vi "DAQ_CounterTrigger_DO_AO_2DAQ.vi"(8 "error in (no error)":errorcluster) -> (0 "error out":errorcluster)   [LabVIEW 2025]
uses:
  SubVIs/State_Machine_Ctrl.ctl
  <vilib>/DAQmx/write.llb/DAQmx Write (Digital 1D Wfm NChan NSamp).vi
  <vilib>/DAQmx/write.llb/DAQmx Write (Analog 1D Wfm NChan NSamp).vi
  <vilib>/Waveform/DWDTOps.llb/DWDT Uncompress Digital.vi
  <vilib>/DAQmx/miscellaneous.llb/DAQmx Fill In Error Info.vi
  <resource>/objmgr/daqmx.rc
panel:
  in  "Z":bool=TRUE
  in  "AO Z":tag="USB-6211/ao1"
  out "AO WF":waveform(dbl)[](graph)=[{"t0"=timestamp(0 s since 1904-01-01), "dt"=0.0001, "Y"=array[9000 elements]}, {"t0"=timestamp(0 s since 1904-01-01), "dt"=0.0001, "Y"=array[9000 elements]}, {"t0"=timestamp(0 s since 1904-01-01), "dt"=0.0001, "Y"=array[9000 elements]}, {"t0"=timestamp(0 s since 1904-01-01), "dt"=0.0001, "Y"=array[9000 elements]}]
  out "DO WF":digitalwaveform[](graph)=[{"t0"=timestamp(0 s since 1904-01-01), "dt"=0.0001, "Y"={"transitions"=[], "data"=array9000x1[9000 elements]}}, {"t0"=timestamp(0 s since 1904-01-01), "dt"=0.0001, "Y"={"transitions"=[], "data"=array9000x1[9000 elements]}}, {"t0"=timestamp(0 s since 1904-01-01), "dt"=0.0001, "Y"={"transitions"=[], "data"=array9000x1[9000 elements]}}, {"t0"=timestamp(0 s since 1904-01-01), "dt"=0.0001, "Y"={"transitions"=[], "data"=array9000x1[9000 elements]}}]
  in  "Polar | ON/OFF":bool=TRUE
  in  "AO | %":dbl[](array[slide])=[9.734513274336283, 23.008849557522126, 41.5929203539823, 65.48672566371681] min=0.0 max=100.0 step=1.0 scale=0.0..100.0
  in  "AO | ON/OFF":bool[](array[boolean])=[TRUE, TRUE, TRUE, TRUE]
  in  "AO Laser":tag="USB-6363/ao0:3"
  in  "AO pockels":tag="USB-6211/ao0"
  in  "DO | ON/OFF":bool[](array[boolean])=[TRUE, TRUE, TRUE, TRUE, TRUE]
  in  "Pre-activation time (s)":dbl=0.03
  in  "Start":bool
  in  "Timing source":tag="OnboardClock"
  in  "Readout time (s)":dbl=0.02
  in  "Exposure time (s)":dbl=0.05
  in  "DO":tag="USB-6363/port0/line0:4"
  in  "Counter":tag="USB-6363/ctr0"
  in  "Stop":bool
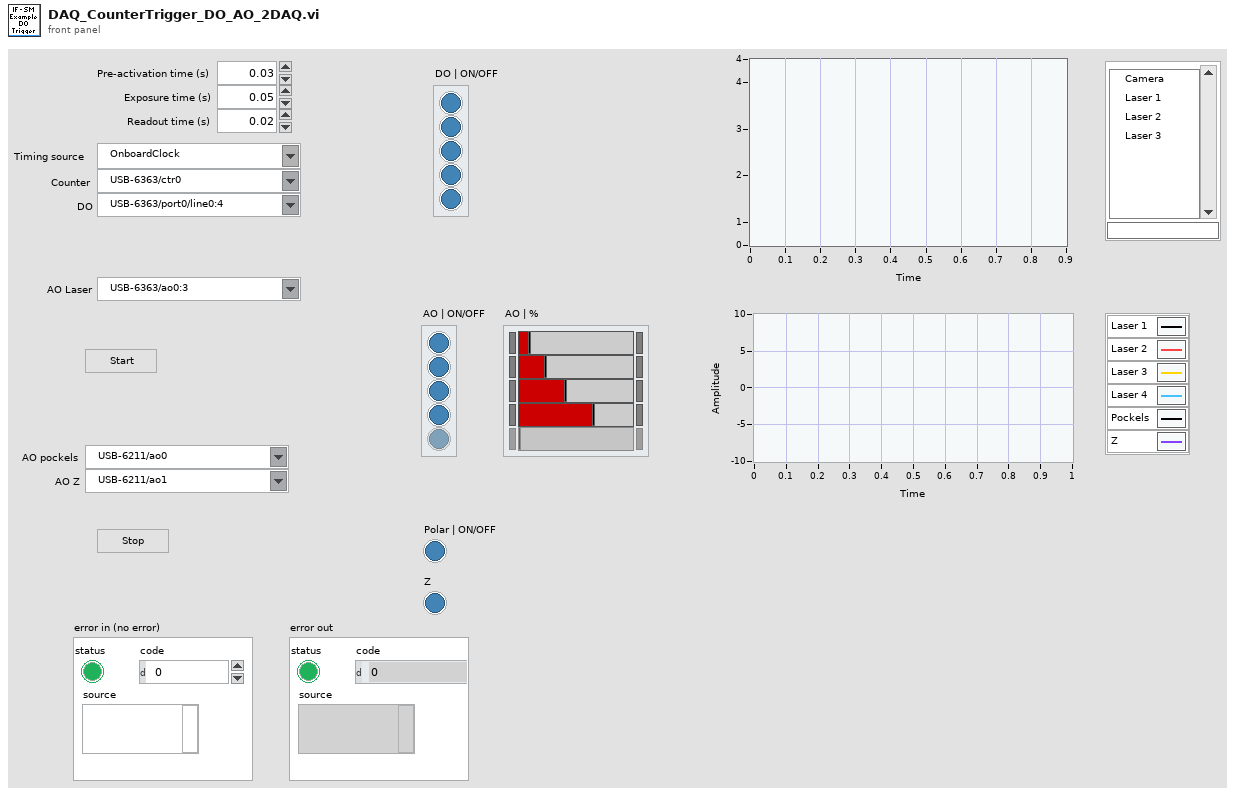
[diagram p1: front panel]
types:
  T1 = typedef "State_Machine_Ctrl.ctl" = enum16{"Initialize", "Wait for Event", "Setup_DAQ", "Create WF", "Generate WF", "Stop"}
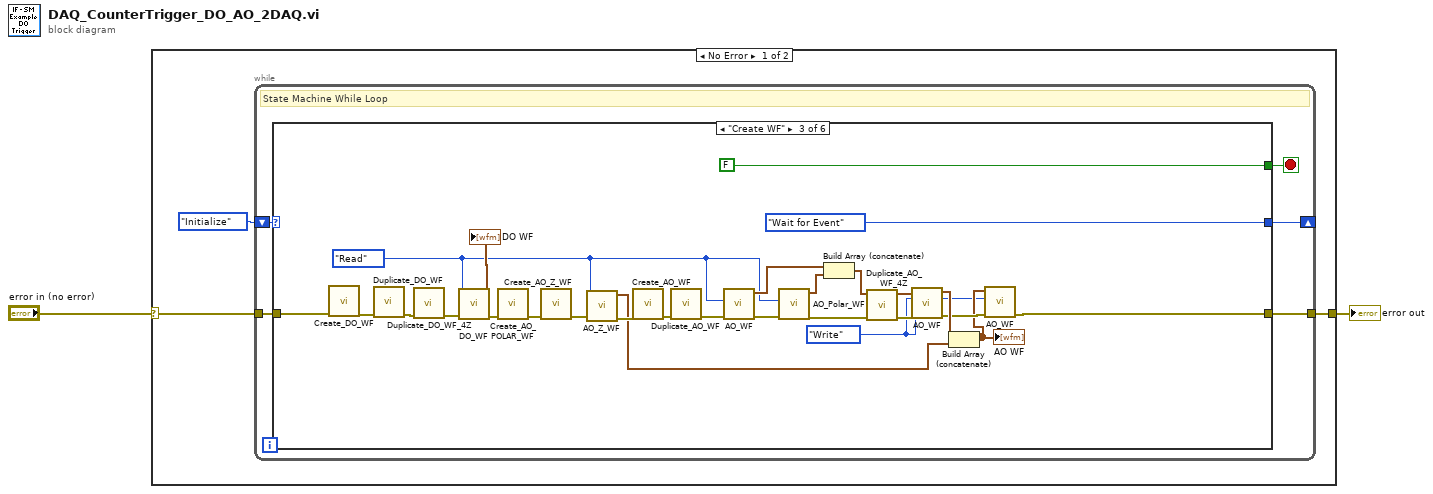
[diagram p0: block diagram]
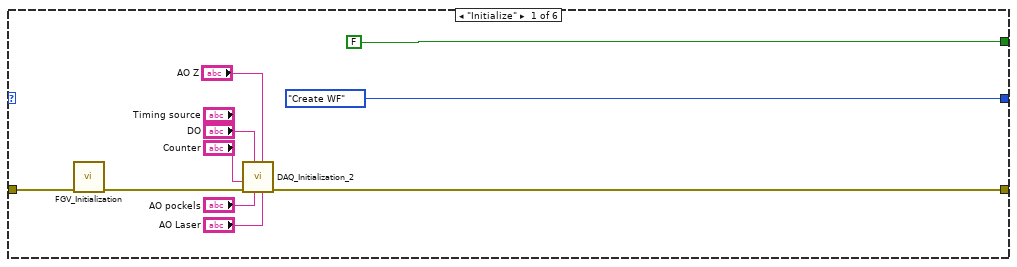
[diagram p2: hidden frame]
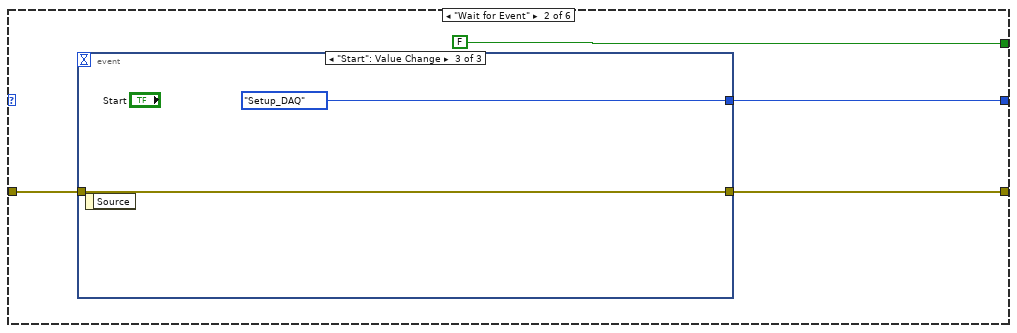
[diagram p3: hidden frame]
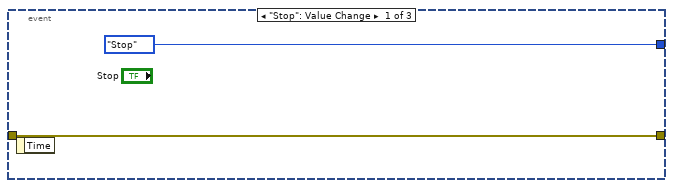
[diagram p4: hidden frame]
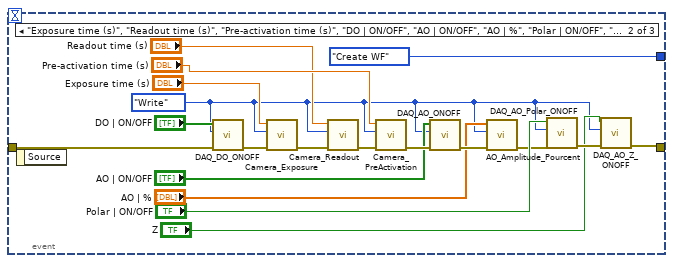
[diagram p5: hidden frame]
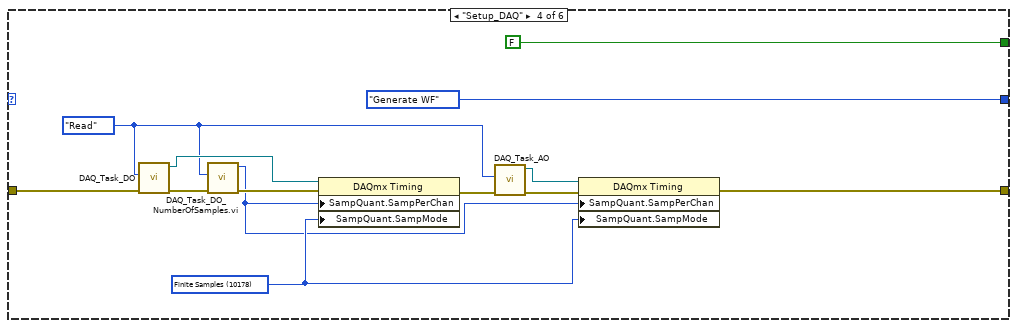
[diagram p6: hidden frame]
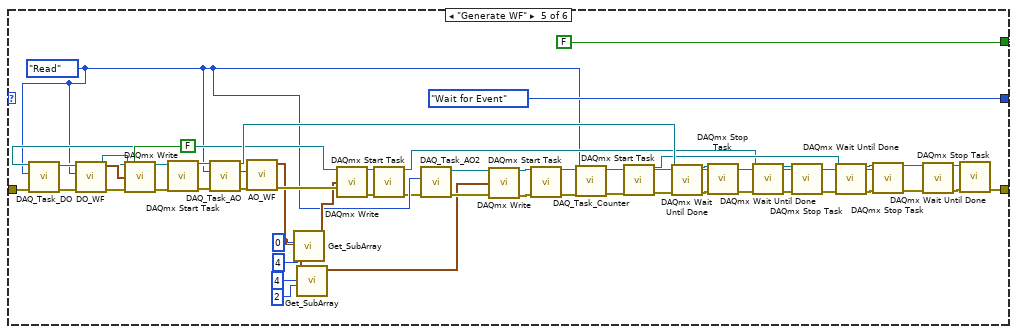
[diagram p7: hidden frame]
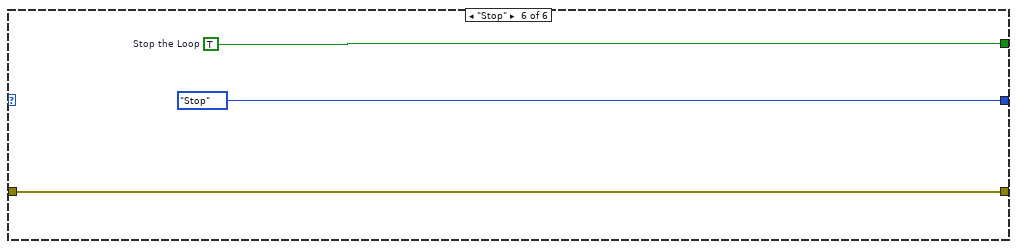
[diagram p8: hidden frame]
diagram:
  n1 = case shown="No Error" "error in (no error)" {
    selector: "error in (no error)" -> [w4 w140]
    tunnel: [w3 w140] -> w2
    frame No Error {
      n2 = while {
        shift-right: [w9] -> _
        shift-left: State_Machine_Ctrl."Initialize" ("Initial State") -> [w10]
        tunnel: w4 -> [w7]
        tunnel: [w6] -> w3
        stop <- w8 stop-if-true
        # "State Machine While Loop"
        n3 = case "State Machine Case Structure" shown="\"Create WF\"" w10 {
          tunnel: [State_Machine_Ctrl."Create WF" ("Initial State") w24 State_Machine_Ctrl."Wait for Event" ("Initial State") State_Machine_Ctrl."Generate WF" ("Initial State") State_Machine_Ctrl."Wait for Event" ("Initial State") State_Machine_Ctrl."Stop" ("Initial State")] -> w9
          tunnel: [FALSE ("Stop the Loop") FALSE ("Stop the Loop") FALSE ("Stop the Loop") FALSE ("Stop the Loop") FALSE ("Stop the Loop") w139] -> w8
          tunnel: w7 -> [w18 w22 w72 w85 w133 w137]
          tunnel: [w19 w21 w50 w82 w107 w137] -> w6
          frame "Initialize" {
            # "Initialize - In this example, the only initialization required is to specify that the next state for the state machine is \"Wait for Event\"."
            n4 = call "FGV_Initialization.vi"("error in (no error)"=w18) -> ("error out"=w17:errorcluster)  [unwired: 10 in]
            n5 = call "DAQ_Initialization_2.vi"("AO Lasers"="AO Laser", "AO Z"="AO Z", "AO Pockels"="AO pockels", "DO"="DO", "error in (no error)"=w17, "Counter"="Counter") -> ("error out"=w19:errorcluster)  [unwired: 5 in]
          }
          frame "Wait for Event" {
            # "Wait for Event - An Event Structure is used to monitor the user interface for events. In each frame of the Event Structure, the next state of the state machine is specified based on which button was pressed."
            n6 = event shown="[2] \"Start\": Value Change" {
              selector: _ -> [_ _ _]
              dyn-events: _ -> [_ _ _]
              timeout: _ -> [_ _ _]
              tunnel: [State_Machine_Ctrl."Stop" ("Initial State") State_Machine_Ctrl."Create WF" ("Initial State") State_Machine_Ctrl."Setup_DAQ" ("Initial State")] -> w24
              tunnel: w22 -> [w25 w41 w46]
              tunnel: [w25 w29 w46] -> w21
              event "Stop": Value Change {
                n7 = event-data() -> ()  [unwired: 1 in, 1 out]
              }
              event "Exposure time (s)", "Readout time (s)", "Pre-activation time (s)", "DO | ON/OFF", "AO | ON/OFF", "AO | %", "Polar | ON/OFF", "Z": Value Change {
                w27 = enum16{"Write", "Read"}."Write" ("Action")
                n8 = event-data() -> ()  [unwired: 1 in, 1 out]
                n9 = call "DAQ_DO_ONOFF.vi"("error in"=w41, "Action"=w27, "DO | ON/OFF"="DO | ON/OFF") -> ("error out"=w44:errorcluster)  [unwired: 7 in, 1 out]
                n10 = call "Camera_Exposure.vi"("error in"=w44, "Action"=w27, "Exposure (s)"="Exposure time (s)") -> ("error out"=w43:errorcluster)  [unwired: 7 in, 1 out]
                n11 = call "Camera_Readout.vi"("error in"=w43, "Action"=w27, "Camera_Readout"="Readout time (s)") -> ("error out"=w42:errorcluster)  [unwired: 7 in, 1 out]
                n12 = call "Camera_PreActivation.vi"("error in"=w42, "Action"=w27, "Camera_PreActivation"="Pre-activation time (s)") -> ("error out"=w36:errorcluster)  [unwired: 7 in, 1 out]
                n13 = call "DAQ_AO_ONOFF.vi"("error in"=w36, "Action"=w27, "AO | ON/OFF"="AO | ON/OFF") -> ("error out"=w34:errorcluster)  [unwired: 7 in, 1 out]
                n14 = call "AO_Amplitude_Pourcent.vi"("error in"=w34, "Action"=w27, "AO | %"="AO | %") -> ("error out"=w31:errorcluster)  [unwired: 7 in, 1 out]
                n15 = call "DAQ_AO_Polar_ONOFF.vi"("error in"=w31, "Action"=w27, "ON / OFF"="Polar | ON/OFF") -> ("error out"=w30:errorcluster)  [unwired: 7 in, 1 out]
                n16 = call "DAQ_AO_Z_ONOFF.vi"("error in"=w30, "Action"=w27, "ON / OFF"="Z") -> ("error out"=w29:errorcluster)  [unwired: 7 in, 1 out]
              }
              event "Start": Value Change {
                n17 = event-data() -> ()  [unwired: 1 in, 1 out]
              }
            }
          }
          frame "Create WF" {
            w48 = enum16{"Write", "Read"}."Write" ("Action")
            w63 = enum16{"Write", "Read"}."Read" ("Action")
            n18 = call "Create_DO_WF.vi"("error in"=w72) -> ("error out"=w71:errorcluster)  [unwired: 10 in]
            n19 = call "Duplicate_DO_WF.vi"("error in"=w71) -> ("error out"=w60:errorcluster)  [unwired: 10 in]
            n20 = call "Duplicate_DO_WF_4Z.vi"("error in"=w60) -> ("error out"=w59:errorcluster)  [unwired: 10 in]
            n21 = call "DO_WF.vi"("error in"=w59, "Action"=w63) -> ("error out"=w58:errorcluster, "Digital WF"=→"DO WF":digitalwaveform[])  [unwired: 8 in]
            n22 = call "Create_AO_POLAR_WF.vi"("error in"=w58) -> ("error out"=w64:errorcluster)  [unwired: 10 in]
            n23 = call "Create_AO_Z_WF.vi"("error in"=w64) -> ("error out"=w62:errorcluster)  [unwired: 10 in]
            n24 = call "AO_Z_WF.vi"("error in"=w62, "Action"=w63) -> ("error out"=w61:errorcluster, "AO Z WF"=w53:waveform(dbl))  [unwired: 8 in]
            n25 = call "Create_AO_WF.vi"("error in"=w61) -> ("error out"=w69:errorcluster)  [unwired: 10 in]
            n26 = call "Duplicate_AO_WF.vi"("error in (no error)"=w69) -> ("error out"=w68:errorcluster)  [unwired: 10 in]
            n27 = call "AO_WF.vi"("error in"=w68, "Action"=w63) -> ("error out"=w70:errorcluster, "AO WF"=w66:waveform(dbl)[])  [unwired: 8 in]
            n28 = call "AO_Polar_WF.vi"("error in"=w70, "Action"=w63) -> ("error out"=w54:errorcluster, "AO Poalr WF"=w65:waveform(dbl))  [unwired: 8 in]
            n29 = Build Array (concatenate)(w66, w65) -> (w57:waveform(dbl)[])
            n30 = call "Duplicate_AO_WF_4Z.vi"("error in (no error)"=w54, "AO WF"=w57) -> ("error out"=w55:errorcluster, "AO WF 2"=w56:waveform(dbl)[])  [unwired: 8 in]
            n31 = call "AO_WF.vi"("error in"=w55, "Action"=w48, "AO WF"=w56) -> ("error out"=w51:errorcluster, "AO WF"=w52:waveform(dbl)[])  [unwired: 7 in]
            n32 = Build Array (concatenate)(w52, w53) -> (w49:waveform(dbl)[])
            "AO WF" <- w49
            n33 = call "AO_WF.vi"("error in"=w51, "Action"=w48, "AO WF"=w49) -> ("error out"=w50:errorcluster)  [unwired: 7 in, 1 out]
          }
          frame "Setup_DAQ" {
            w79 = 10178 items=["Finite Samples"=10178, "Continuous Samples"=10123, "Hardware Timed Single Point"=12522] ("SampQuant.SampMode")
            w78 = enum16{"Write", "Read"}."Read" ("Action")
            n34 = call "DAQ_Task_DO.vi"("error in"=w85, "Action"=w78) -> ("error out"=w77:errorcluster, "DAQ_Task_DO"=w84:refnum<k21>)  [unwired: 8 in]
            n35 = call "DAQ_Task_DO_NumberOfSamples.vi.vi"("error in"=w77, "Action"=w78) -> ("error out"=w76:errorcluster, "Samples"=w75:u32)  [unwired: 8 in]
            n36 = property class="DAQmx Timing"(reference=w84, error in=w76, "SampQuant.SampPerChan"=w75, "SampQuant.SampMode"=w79) -> (error out=w80:errorcluster)  [unwired: 1 out]
            n37 = call "DAQ_Task_AO.vi"("error in"=w80, "Action"=w78) -> ("error out"=w83:errorcluster, "DAQ_Task_AO"=w81:refnum<k21>)  [unwired: 8 in]
            n38 = property class="DAQmx Timing"(reference=w81, error in=w83, "SampQuant.SampPerChan"=w75, "SampQuant.SampMode"=w79) -> (error out=w82:errorcluster)  [unwired: 1 out]
          }
          frame "Generate WF" {
            w97 = enum16{"Write", "Read"}."Read" ("Action")
            n39 = call "DAQ_Task_DO.vi"("error in"=w133, "Action"=w97) -> ("error out"=w120:errorcluster, "DAQ_Task_DO"=w132:refnum<k21>)  [unwired: 8 in]
            n40 = call "DO_WF.vi"("error in"=w120, "Action"=w97) -> ("error out"=w119:errorcluster, "Digital WF"=w121:digitalwaveform[])  [unwired: 8 in]
            n41 = call-poly <vilib>:"DAQmx Write.vi"("task/channels in"=w132, "auto start"=FALSE, "data"=w121, "error in"=w119) -> ("task out"=w131:refnum<k21>, "error out"=w134:errorcluster)  [unwired: 9 in, 1 out]
            n42 = call <vilib>:"DAQmx Start Task.vi"("task/channels in"=w131, "error in"=w134) -> ("task out"=w125:refnum<k21>, "error out"=w101:errorcluster)  [unwired: 12 in]
            n43 = call "DAQ_Task_AO.vi"("error in"=w101, "Action"=w97) -> ("error out"=w114:errorcluster, "DAQ_Task_AO"=w113:refnum<k21>)  [unwired: 8 in]
            n44 = call "AO_WF.vi"("error in"=w114, "Action"=w97) -> ("error out"=w112:errorcluster, "AO WF"=w91:waveform(dbl)[])  [unwired: 8 in]
            n45 = call "Get_SubArray.vi"("length"=4, "index"=0, "AO WF"=w91) -> ("Sub array"=w99:waveform(dbl)[])  [unwired: 8 in]
            n46 = call "Get_SubArray.vi"("length"=2, "index"=4, "AO WF"=w91) -> ("Sub array"=w90:waveform(dbl)[])  [unwired: 8 in]
            n47 = call-poly <vilib>:"DAQmx Write.vi"("task/channels in"=w113, "data"=w99, "error in"=w112) -> ("task out"=w111:refnum<k21>, "error out"=w110:errorcluster)  [unwired: 10 in, 1 out]
            n48 = call <vilib>:"DAQmx Start Task.vi"("task/channels in"=w111, "error in"=w110) -> ("task out"=w109:refnum<k21>, "error out"=w94:errorcluster)  [unwired: 12 in]
            n49 = call "DAQ_Task_AO2.vi"("error in"=w94, "Action"=w97) -> ("error out"=w100:errorcluster, "DAQ_Task_AO"=w105:refnum<k21>)  [unwired: 8 in]
            n50 = call-poly <vilib>:"DAQmx Write.vi"("task/channels in"=w105, "data"=w90, "error in"=w100) -> ("task out"=w104:refnum<k21>, "error out"=w103:errorcluster)  [unwired: 10 in, 1 out]
            n51 = call <vilib>:"DAQmx Start Task.vi"("task/channels in"=w104, "error in"=w103) -> ("task out"=w102:refnum<k21>, "error out"=w95:errorcluster)  [unwired: 12 in]
            n52 = call "DAQ_Task_Counter.vi"("error in"=w95, "Action"=w97) -> ("error out"=w96:errorcluster, "DAQ_Task_Counter"=w130:refnum<k21>)  [unwired: 8 in]
            n53 = call <vilib>:"DAQmx Start Task.vi"("task/channels in"=w130, "error in"=w96) -> ("task out"=w123:refnum<k21>, "error out"=w122:errorcluster)  [unwired: 12 in]
            n54 = call <vilib>:"DAQmx Wait Until Done.vi"("task/channels in"=w125, "error in"=w122) -> ("task out"=w124:refnum<k21>, "error out"=w126:errorcluster)  [unwired: 12 in]
            n55 = call <vilib>:"DAQmx Stop Task.vi"("task/channels in"=w124, "error in"=w126) -> ("error out"=w117:errorcluster)  [unwired: 12 in, 1 out]
            n56 = call <vilib>:"DAQmx Wait Until Done.vi"("task/channels in"=w109, "error in"=w117) -> ("task out"=w115:refnum<k21>, "error out"=w118:errorcluster)  [unwired: 12 in]
            n57 = call <vilib>:"DAQmx Stop Task.vi"("task/channels in"=w115, "error in"=w118) -> ("error out"=w116:errorcluster)  [unwired: 12 in, 1 out]
            n58 = call <vilib>:"DAQmx Wait Until Done.vi"("task/channels in"=w123, "error in"=w116) -> ("task out"=w128:refnum<k21>, "error out"=w127:errorcluster)  [unwired: 12 in]
            n59 = call <vilib>:"DAQmx Stop Task.vi"("task/channels in"=w128, "error in"=w127) -> ("error out"=w106:errorcluster)  [unwired: 12 in, 1 out]
            n60 = call <vilib>:"DAQmx Wait Until Done.vi"("task/channels in"=w102, "error in"=w106) -> ("task out"=w98:refnum<k21>, "error out"=w108:errorcluster)  [unwired: 12 in]
            n61 = call <vilib>:"DAQmx Stop Task.vi"("task/channels in"=w98, "error in"=w108) -> ("error out"=w107:errorcluster)  [unwired: 12 in, 1 out]
          }
          frame "Stop" {
            w139 = TRUE  # Stop the Loop
            # "Stop - Stop the VI. This is the only state that specifies a TRUE value for the loop conditional terminal."
          }
        }
      }
    }
    frame Error {
    }
  }
  "error out" <- w2
